vi "verifySignatureIntegers.vi"(6 "timeout (10000)":i32=10000, 8 "error in (no error)":errorcluster, 11 "Request":T1={"random"={"method"="", "hashedApiKey"="", "n"=0, "min"=0, "max"=0, "replacement"=TRUE, "base"=10, "data"=[], "completionTime"="", "serialNumber"=0}, "signature"="", "id"=0.0} {"random"."base" items=["2"=2, "8"=8, "10"=10, "16"=16]}) -> (0 "error out":errorcluster, 3 "Response":T2, 4 "error data":string[](array[string]))   [LabVIEW 2014, in "Random JSON API.lvlib"]
uses:
  Random JSON API.lvlib
  Type Defs/verifySignatureResponse.ctl
  Type Defs/verifySignatureIntegersRequest.ctl
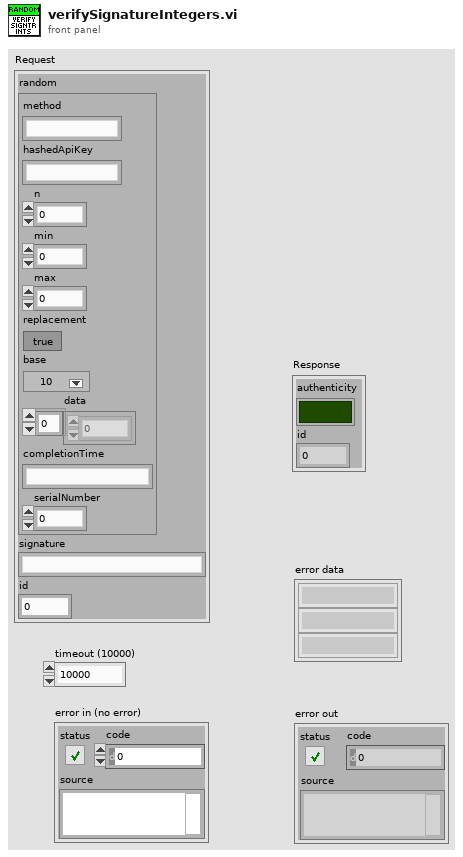
[diagram p1: front panel]
types:
  T1 = typedef "Random JSON API.lvlib/verifySignatureIntegersRequest.ctl" = cluster{"random":cluster{"method":string, "hashedApiKey":string, "n":i32, "min":i32, "max":i32, "replacement":bool, "base":i32, "data":i32[], "completionTime":string, "serialNumber":i32}, "signature":string, "id":dbl}
  T2 = typedef "Random JSON API.lvlib/verifySignatureResponse.ctl" = cluster{"authenticity":bool, "id":dbl}
  T3 = cluster{"jsonrpc":string, "method":string, "params":cluster{"random":cluster{"method":string, "hashedApiKey":string, "n":i32, "min":i32, "max":i32, "replacement":bool, "base":i32, "data":i32[], "completionTime":string, "serialNumber":i32}, "signature":string}, "id":dbl}
  T4 = cluster{"jsonrpc":string, "method":string, "params":cluster{"random":cluster{"method":string, "hashedApiKey":string, "n":i32, "min":i32, "max":i32, "replacement":bool, "base":i32, "data":string[], "completionTime":string, "serialNumber":i32}, "signature":string}, "id":dbl}
  T5 = cluster{"method":string, "hashedApiKey":string, "n":i32, "min":i32, "max":i32, "replacement":bool, "base":i32, "data":i32[], "completionTime":string, "serialNumber":i32}
  T6 = cluster{cluster{"method":string, "hashedApiKey":string, "n":i32, "min":i32, "max":i32, "replacement":bool, "base":i32, "data":i32[], "completionTime":string, "serialNumber":i32}, "signature":string}
  T7 = cluster{"method":string, "hashedApiKey":string, "n":i32, "min":i32, "max":i32, "replacement":bool, "base":i32, string[], "completionTime":string, "serialNumber":i32}
  T8 = cluster{cluster{"method":string, "hashedApiKey":string, "n":i32, "min":i32, "max":i32, "replacement":bool, "base":i32, string[], "completionTime":string, "serialNumber":i32}, "signature":string}
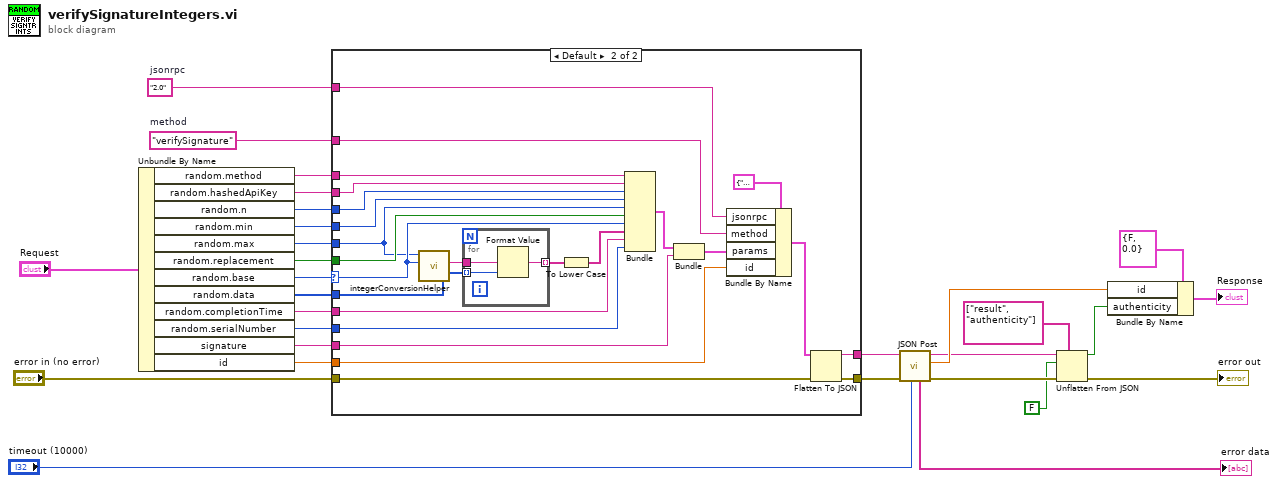
[diagram p0: block diagram]
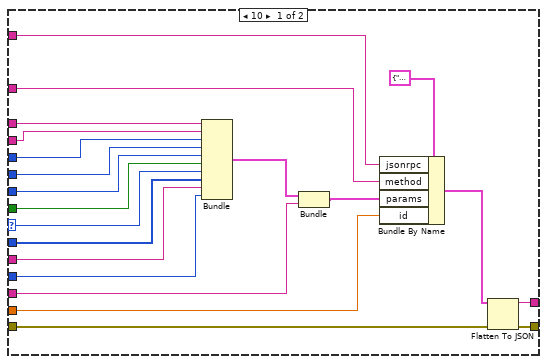
[diagram p2: hidden frame]
diagram:
  w6 = "2.0"  # jsonrpc
  w7 = "verifySignature"  # method
  n1 = Unbundle By Name("Request") -> ("random.method"=w8:string, "random.hashedApiKey"=w9:string, "random.n"=w10:i32, "random.min"=w11:i32, "random.max"=w12:i32, "random.replacement"=w13:bool, "random.base"=w19:i32, "random.data"=w18:i32[], "random.completionTime"=w17:string, "random.serialNumber"=w16:i32, "signature"=w15:string, "id"=w14:dbl)
  n2 = case shown="Default" w19 {
    selector: w19 -> [w36 w57]
    tunnel: w18 -> [w35 w54]
    tunnel: w17 -> [w34 w63]
    tunnel: w16 -> [w33 w62]
    tunnel: w15 -> [w44 w69]
    tunnel: w14 -> [w46 w71]
    tunnel: w13 -> [w37 w64]
    tunnel: w12 -> [w38 w56]
    tunnel: w11 -> [w39 w65]
    tunnel: w10 -> [w40 w66]
    tunnel: w9 -> [w41 w67]
    tunnel: w8 -> [w42 w68]
    tunnel: w7 -> [w47 w72]
    tunnel: w6 -> [w48 w73]
    tunnel: "error in (no error)" -> [w32 w61]
    tunnel: [w31 w60] -> w4
    tunnel: [w30 w59] -> w3
    frame 10 {
      n3 = Bundle("method"=w42, "hashedApiKey"=w41, "n"=w40, "min"=w39, "max"=w38, "replacement"=w37, "base"=w36, "data"=w35, "completionTime"=w34, "serialNumber"=w33) -> (w45:T5)  [unwired: 1 in]
      n4 = Bundle(w45, "signature"=w44) -> (w43:T6)  [unwired: 1 in]
      n5 = Bundle By Name(cluster=T3 {"jsonrpc"="2.0", "method"="verifySignature", "params"={"random"={"method"="", "hashedApiKey"="", "n"=0, "min"=0, "max"=0, "replacement"=TRUE, "base"=10, "data"=[], "completionTime"="", "serialNumber"=0}, "signature"=""}, "id"=0.0}, "jsonrpc"=w48, "method"=w47, "params"=w43, "id"=w46) -> (w49:T3)
      n6 = Flatten To JSON(anything=w49, error in (no error)=w32) -> (JSON string=w30:string, 11:w31:errorcluster)  [unwired: 1 in]
    }
    frame Default {
      n7 = call "integerConversionHelper.vi"("base"=w57, "max"=w56) -> ("base conversion string"=w53:string)  [unwired: 9 in]
      n8 = for {
        tunnel: w54 -> [w77] mode=indexing
        tunnel: w53 -> [w76]
        tunnel: [w75] -> w52 mode=indexing
        n9 = Format Value(format string=w76, value (0)=w77) -> (output string=w75:string)  [unwired: 1 in]
      }
      n10 = To Lower Case(string=w52) -> (all lower case string=w51:string[])
      n11 = Bundle("method"=w68, "hashedApiKey"=w67, "n"=w66, "min"=w65, "max"=w56, "replacement"=w64, "base"=w57, w51, "completionTime"=w63, "serialNumber"=w62) -> (w70:T7)  [unwired: 1 in]
      n12 = Bundle(w70, "signature"=w69) -> (w55:T8)  [unwired: 1 in]
      n13 = Bundle By Name(cluster=T4 {"jsonrpc"="2.0", "method"="verifySignature", "params"={"random"={"method"="", "hashedApiKey"="", "n"=0, "min"=0, "max"=0, "replacement"=TRUE, "base"=10, "data"=[], "completionTime"="", "serialNumber"=0}, "signature"=""}, "id"=0.0}, "jsonrpc"=w73, "method"=w72, "params"=w55, "id"=w71) -> (w74:T4)
      n14 = Flatten To JSON(anything=w74, error in (no error)=w61) -> (JSON string=w59:string, 11:w60:errorcluster)  [unwired: 1 in]
    }
  }
  n15 = call "JSON Post.vi"("timeout (10000)"="timeout (10000)", "error in (no error)"=w4, "Request JSON String"=w3) -> ("error out"=w26:errorcluster, "id"=w27:dbl, "Response JSON String"=w22:string, "error data"=→"error data":string[])  [unwired: 5 in]
  n16 = Unflatten From JSON(path=string[] ["result", "authenticity"], JSON string=w22, type and defaults=FALSE, error in (no error)=w26) -> (value=w24:bool, error out=→"error out":errorcluster)  [unwired: 3 in]
  n17 = Bundle By Name(cluster=T2 {"authenticity"=FALSE, "id"=0.0} ("Response"), "id"=w27, "authenticity"=w24) -> (→"Response":T2)
